vi "Filter Message Raw.vi"(9 "Excluded Message Types":refnum<class>[](array[class]), 10 "Included Message Types":refnum<class>[](array[class]), 11 "Message in":refnum<class "Message.lvclass">) -> (3 "Checkbox":bool)   [LabVIEW 2020, in "Actor Pub Sub Channels.lvlib" / "Pub Sub Message Channel.lvclass"]
uses:
  Pub Sub Message Channel.lvclass
  <vilib>/ActorFramework/Message/Message.lvclass
  Pub Sub Message Channel.lvclass/Pub Sub Message Channel.ctl
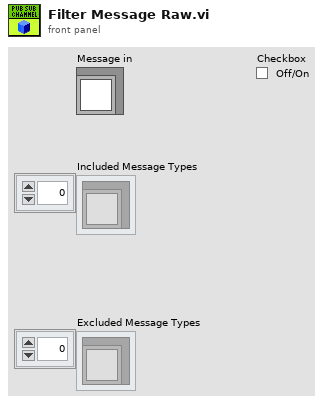
[diagram p1: front panel]
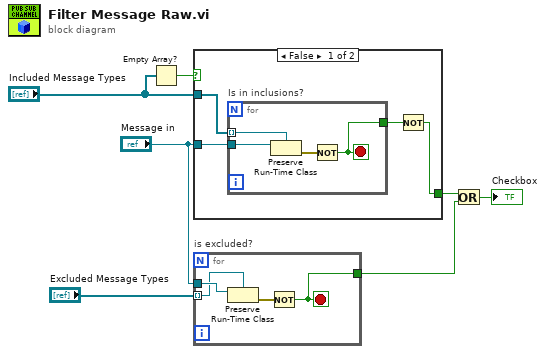
[diagram p0: block diagram]
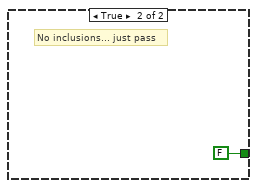
[diagram p2: hidden frame]
diagram:
  n1 = Empty Array?(array="Included Message Types") -> (empty?=w6:bool)
  n2 = case shown="False" w6 {
    tunnel: "Included Message Types" -> [w11 _]
    tunnel: [w9 FALSE] -> w5
    tunnel: "Message in" -> [w10 _]
    frame False {
      n3 = for "Is in inclusions?" {
        tunnel: w11 -> [w14] mode=indexing
        tunnel: w10 -> [w15]
        tunnel: [w12] -> w8
        stop <- w12 stop-if-true
        n4 = Preserve Run-Time Class(object in=w15, 2:w14) -> (error out=w13:errorcluster)  [unwired: 1 in, 1 out]
        n5 = Not(x=w13) -> (.not. x?=w12:bool)
      }
      n6 = Not(x=w8) -> (.not. x?=w9:bool)
    }
    frame True {
      # "No inclusions... just pass"
    }
  }
  n7 = for "is excluded?" {
    tunnel: "Excluded Message Types" -> [w19] mode=indexing
    tunnel: "Message in" -> [w20]
    tunnel: [w17] -> w1
    stop <- w17 stop-if-true
    n8 = Preserve Run-Time Class(object in=w20, 2:w19) -> (error out=w18:errorcluster)  [unwired: 1 in, 1 out]
    n9 = Not(x=w18) -> (.not. x?=w17:bool)
  }
  n10 = Or(x=w5, y=w1) -> (x .or. y?=→"Checkbox":bool)
